vi "Get Panel Hwnd.vi"(8 "error in (no error)":errorcluster, 11 "Panel":refnum<k24>(container)) -> (0 "error out":errorcluster, 2 "HWND":i32, 3 "Container reference out":refnum<k24>)   [LabVIEW 2016, in "LV MDI.lvclass"]
doc: "Get MDI panel Hwnd."
uses:
  LV MDI.lvclass
  System.Windows.Forms
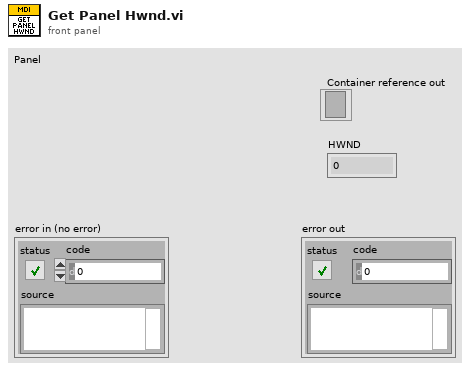
[diagram p1: front panel]
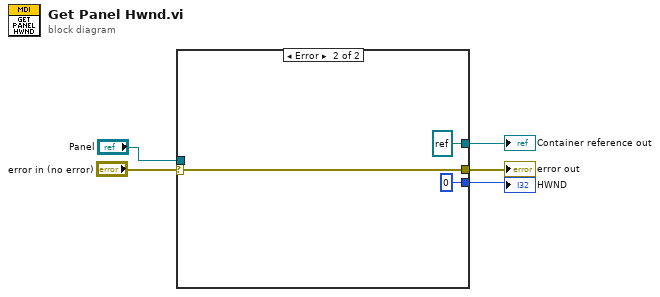
[diagram p0: block diagram]
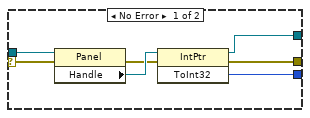
[diagram p2: hidden frame]
diagram:
  n1 = case shown="Error" "error in (no error)" {
    selector: "error in (no error)" -> [w7 w14]
    tunnel: [w10 refnum<k24> refnum ("Handle")] -> w5
    tunnel: [w9 w14] -> w4
    tunnel: [w8 0 ("ToInt64")] -> w3
    tunnel: "Panel" -> [w6 _]
    frame No Error {
      n2 = property class="Panel"(reference=w6, error in=w7) -> (error out=w11:errorcluster, "Handle"=w12:refnum<k24>)  [unwired: 1 out]
      n3 = invoke class="IntPtr" method="ToInt32"(reference=w12, error in=w11) -> (reference out=w10:refnum<k24>, error out=w9:errorcluster, "ToInt32"=w8:i32)  [unwired: 1 in]
    }
    frame Error {
    }
  }
  "Container reference out" <- w5
  "error out" <- w4
  "HWND" <- w3
